vi "ButtonCycle.vi"(8 "Start At":i32, 9 "MaxNum":i32, 10 "FlashInput":bool) -> (2 "CycleNumber":i32)   [LabVIEW 2020]
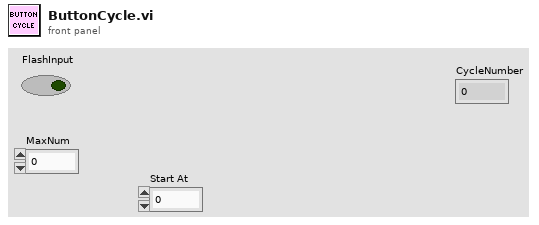
[diagram p1: front panel]
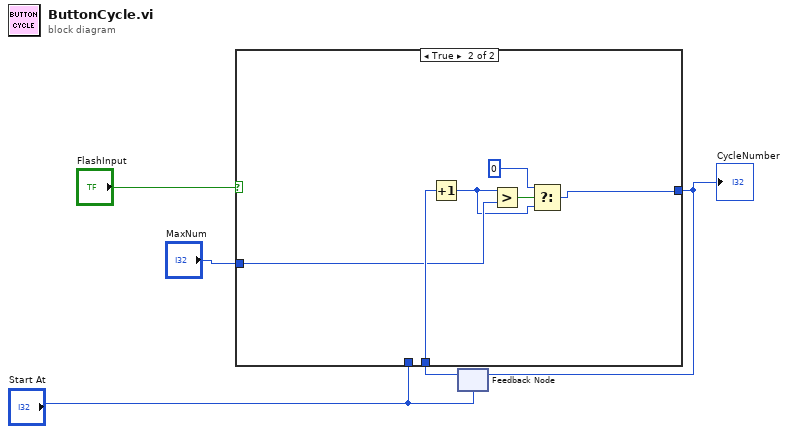
[diagram p0: block diagram]
diagram:
  n1 = feedback #1("Start At") -> (w3:i32)
  n2 = case shown="True" "FlashInput" {
    tunnel: [w6 w7] -> w4
    tunnel: w3 -> [w6 w12]
    tunnel: "Start At" -> [_ _]
    tunnel: "MaxNum" -> [_ w10]
    frame False {
    }
    frame True {
      n3 = Increment(x=w12) -> (x+1=w8:i32)
      n4 = Greater?(x=w8, y=w10) -> (0:w11:bool)
      n5 = Select(t=0, s=w11, f=w8) -> (s? t:f=w7:i32)
    }
  }
  "CycleNumber" <- w4
  n6 = feedback-in #1(w4) -> ()
